vi "SSC DCPower Force Voltage Array Asymmetric Limits.vi"(0 "DCPower SSC in":T1[](array[typedef]), 1 "Voltage Level Range (V)":dbl[](array[numeric]) format="%#_6p", 2 "Current Limit Range (A)":dbl[](array[numeric]) format="%#_6p", 5 "Voltage Level (V)":dbl[](array[numeric]) format="%#_6p", 7 "Current Limit High (A)":dbl[](array[numeric]) format="%#_6p", 9 "Current Limit Low (A)":dbl[](array[numeric]) format="%#_6p", 11 "error in":errorcluster) -> (4 "DCPower SSC out":T1[](array[typedef]), 15 "error out":errorcluster)   [LabVIEW 2019]
doc: "This VI forces voltage on the provided sessions.\n\nAll input arrays need to be populated with a value for each session, or else the for loop won't iterate for all sessions."
uses:
  SSC DCPower.ctl
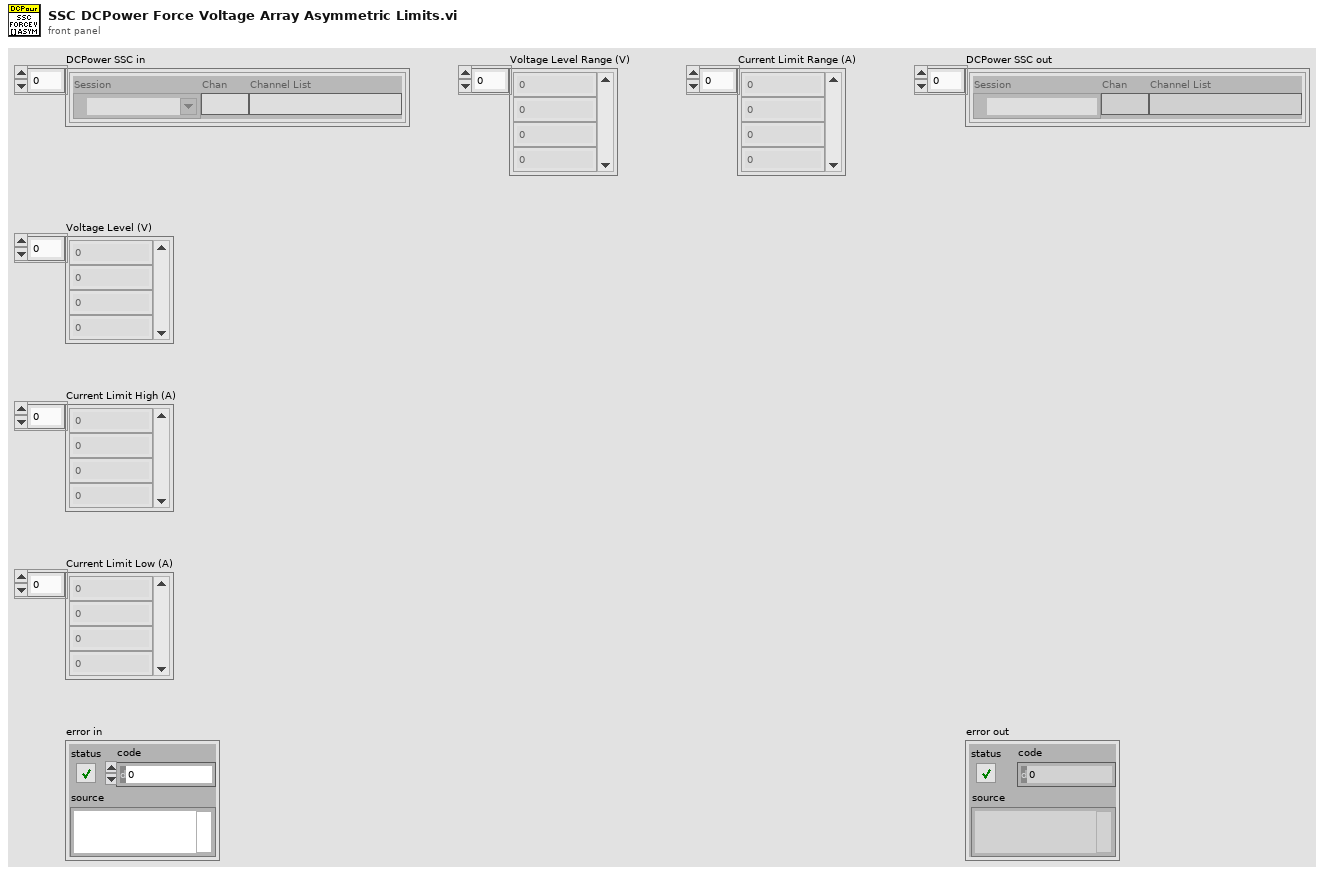
[diagram p1: front panel]
types:
  T1 = typedef "SSC DCPower.ctl" = cluster{"Session":refnum<k15>, "Chan":string, "Channel List":string}
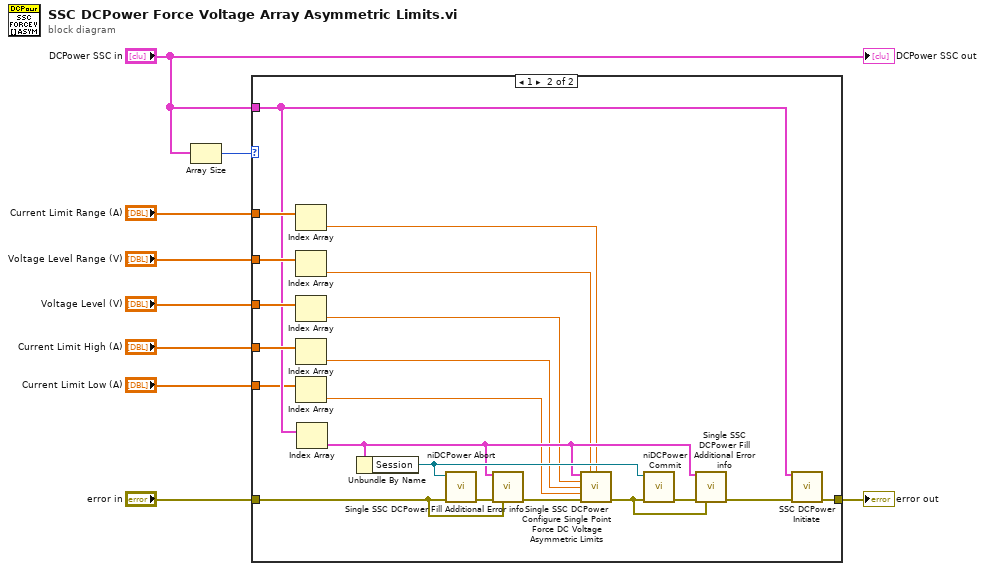
[diagram p0: block diagram]
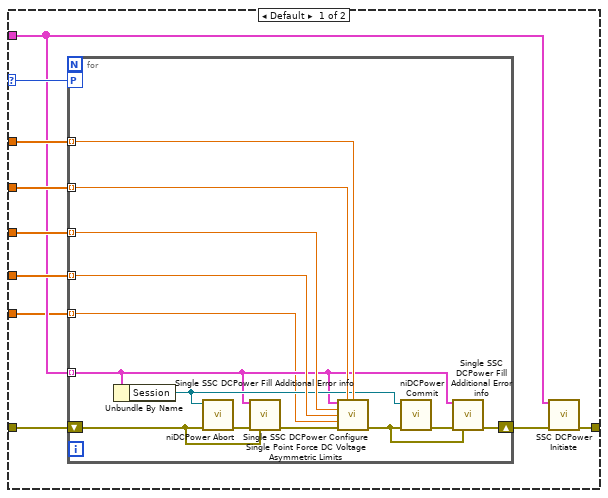
[diagram p2: hidden frame]
diagram:
  n1 = Array Size(array="DCPower SSC in") -> (size(s)=w9:i32)
  n2 = case shown="1" w9 {
    selector: w9 -> [w19 _]
    tunnel: "Voltage Level (V)" -> [w18 w52]
    tunnel: "Current Limit High (A)" -> [w17 w51]
    tunnel: "Voltage Level Range (V)" -> [w16 w50]
    tunnel: [w14 w48] -> w5
    tunnel: "error in" -> [w13 w47]
    tunnel: "Current Limit Range (A)" -> [w12 w46]
    tunnel: "DCPower SSC in" -> [w11 w45]
    tunnel: "Current Limit Low (A)" -> [w10 w34]
    frame Default {
      n3 = for {
        workers-P: w19 -> [_]
        tunnel: w11 -> [w21] mode=indexing
        tunnel: w18 -> [w32] mode=indexing
        tunnel: w17 -> [w31] mode=indexing
        tunnel: w16 -> [w30] mode=indexing
        tunnel: w12 -> [w29] mode=indexing
        shift-right: [w24] -> w15
        shift-left: w13 -> [w23]
        tunnel: w10 -> [w20] mode=indexing
        n4 = Unbundle By Name(w21) -> ("Session"=w26:refnum<k15>)
        n5 = call <instrlib>:"niDCPower Abort.vi"("error in (no error)"=w23, "instrument handle"=w26) -> ("error out"=w28:errorcluster)  [unwired: 8 in, 1 out]
        n6 = call "Single SSC DCPower Fill Additional Error info.vi"("DCPower SSC in"=w21, "error in"=w28, "previous error in"=w23) -> ("error out"=w25:errorcluster)  [unwired: 12 in]
        n7 = call "Single SSC DCPower Configure Single Point Force DC Voltage Asymmetric Limits.vi"("DCPower SSC in"=w21, "Voltage Level Range (V)"=w30, "Current Limit Range (A)"=w29, "Voltage Level (V)"=w32, "Current Limit High (A)"=w31, "Current Limit Low (A)"=w20, "error in"=w25) -> ("error out"=w22:errorcluster)  [unwired: 7 in, 1 out]
        n8 = call <instrlib>:"niDCPower Commit.vi"("error in (no error)"=w22, "instrument handle"=w26) -> ("error out"=w27:errorcluster)  [unwired: 8 in, 1 out]
        n9 = call "Single SSC DCPower Fill Additional Error info.vi"("DCPower SSC in"=w21, "error in"=w27, "previous error in"=w22) -> ("error out"=w24:errorcluster)  [unwired: 12 in]
      }
      n10 = call "SSC DCPower Initiate.vi"("DCPower SSC in"=w11, "error in"=w15) -> ("error out"=w14:errorcluster)  [unwired: 12 in, 1 out]
    }
    frame 1 {
      n11 = Index Array(array=w46) -> (element=w38:dbl)  [unwired: 1 in]
      n12 = Index Array(array=w50) -> (element=w37:dbl)  [unwired: 1 in]
      n13 = Index Array(array=w52) -> (element=w36:dbl)  [unwired: 1 in]
      n14 = Index Array(array=w51) -> (element=w35:dbl)  [unwired: 1 in]
      n15 = Index Array(array=w34) -> (element=w33:dbl)  [unwired: 1 in]
      n16 = Index Array(array=w45) -> (element=w39:T1)  [unwired: 1 in]
      n17 = Unbundle By Name(w39) -> ("Session"=w42:refnum<k15>)
      n18 = call <instrlib>:"niDCPower Abort.vi"("error in (no error)"=w47, "instrument handle"=w42) -> ("error out"=w44:errorcluster)  [unwired: 8 in, 1 out]
      n19 = call "Single SSC DCPower Fill Additional Error info.vi"("DCPower SSC in"=w39, "error in"=w44, "previous error in"=w47) -> ("error out"=w41:errorcluster)  [unwired: 12 in]
      n20 = call "Single SSC DCPower Configure Single Point Force DC Voltage Asymmetric Limits.vi"("DCPower SSC in"=w39, "Voltage Level Range (V)"=w37, "Current Limit Range (A)"=w38, "Voltage Level (V)"=w36, "Current Limit High (A)"=w35, "Current Limit Low (A)"=w33, "error in"=w41) -> ("error out"=w40:errorcluster)  [unwired: 7 in, 1 out]
      n21 = call <instrlib>:"niDCPower Commit.vi"("error in (no error)"=w40, "instrument handle"=w42) -> ("error out"=w43:errorcluster)  [unwired: 8 in, 1 out]
      n22 = call "Single SSC DCPower Fill Additional Error info.vi"("DCPower SSC in"=w39, "error in"=w43, "previous error in"=w40) -> ("error out"=w49:errorcluster)  [unwired: 12 in]
      n23 = call "SSC DCPower Initiate.vi"("DCPower SSC in"=w45, "error in"=w49) -> ("error out"=w48:errorcluster)  [unwired: 12 in, 1 out]
    }
  }
  "error out" <- w5
  "DCPower SSC out" <- "DCPower SSC in"
